vi "Global variable.vi"() -> ()   [LabVIEW 2016]
panel:
  in  "选择区起始":u32
  in  "指令窗":string
  in  "指令集合":string[][](array[string])
  out "error out":errorcluster
  in  "寄存图像":u16[][](array[numeric])
  in  "进度":u8
  in  "I2C_download":bool
  in  "I2C_Download":string
  in  "VISA resource name":refnum<visa-resource-name>
  in  "COM":bool
  # "通用变量"
  # "命令解释器"
  # "I2C_download"
  # "状态量"
  # "图像"
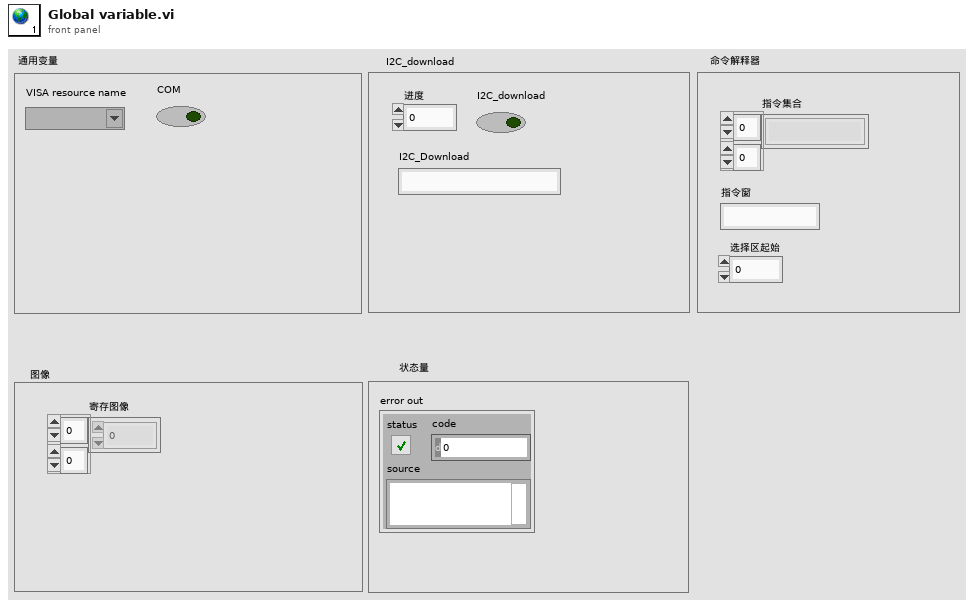
[diagram p1: front panel]
diagram:
